vi "configureTiming.vi"(8 "error in (no error)":errorcluster, 11 "ICCameraAcquisitor in":refnum<class "ICCameraAcquisitor.lvclass">) -> (0 "error out":errorcluster, 3 "ICCameraAcquisitor out":refnum<class "ICCameraAcquisitor.lvclass">)   [LabVIEW 2009, in "Hardware.lvlib" / "Channels.lvlib" / "ICCameraAcquisitor.lvclass"]
uses:
  ICCameraAcquisitor.lvclass
  ICCameraAcquisitor.lvclass/ICCameraAcquisitor.ctl
  CameraAcquisitor.lvclass
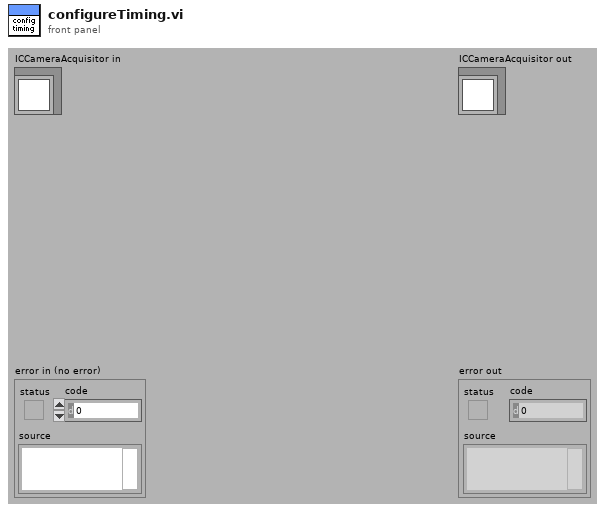
[diagram p1: front panel]
types:
  T1 = cluster{"shutter Open Time":dbl, "Shutter Close Time":dbl, "Exposure Time":dbl, " AccumulatedCycleTime":dbl, " KineticCycleTime":dbl, "Number of Accumulations":dbl, "Number in Kinetic Series ":dbl, "Shutter Mode":dbl}
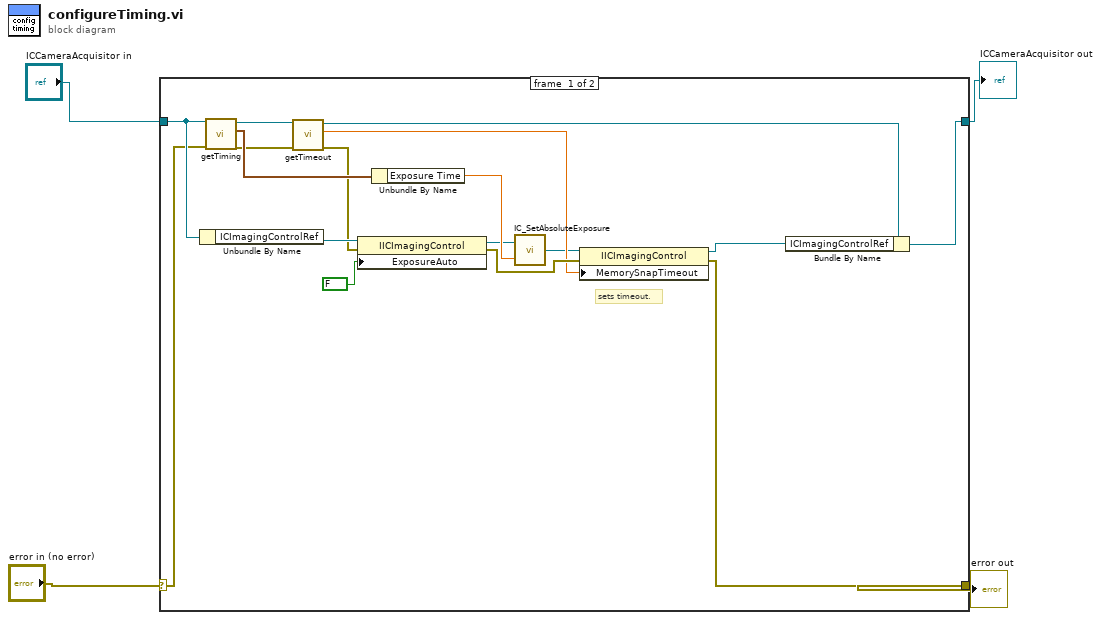
[diagram p0: block diagram]
diagram:
  n1 = case shown="No Error" "error in (no error)" {
    selector: "error in (no error)" -> [w18 w22]
    tunnel: "ICCameraAcquisitor in" -> [w19 w23]
    tunnel: [w10 w23] -> w3
    tunnel: [w14 w22] -> w1
    frame #0 {
      # "sets timeout."
      n2 = Unbundle By Name(w19) -> ("ICImagingControlRef"=w20:refnum<k7>)
      n3 = call-dynamic "getTiming.vi"("error in (no error)"=w18, "CameraAcquisitor.lvclass in"=w19) -> ("error out"=w9:errorcluster, "Timing"=w17:T1, "CameraAcquisitor.lvclass out"=w13:refnum<class "ICCameraAcquisitor.lvclass">)  [unwired: 7 in]
      n4 = call "getTimeout.vi"("error in (no error)"=w9, "CameraAcquisitor.lvclass in"=w13) -> ("error out"=w8:errorcluster, "Timeout"=w12:dbl, "CameraAcquisitor.lvclass out"=w11:refnum<class "ICCameraAcquisitor.lvclass">)  [unwired: 7 in]
      n5 = property class="IICImagingControl"(reference=w20, error in=w8, "ExposureAuto"=FALSE) -> (reference out=w5:refnum<k7>, error out=w15:errorcluster)
      n6 = Unbundle By Name(w17) -> ("Exposure Time"=w7:dbl)
      n7 = call <userlib>:"IC_SetAbsoluteExposure.vi"("Absolute Exposure Time"=w7, "ICImagingControl 4"=w5) -> ("ICImagingControl 3"=w6:refnum<k7>)
      n8 = property class="IICImagingControl"(reference=w6, error in=w15, "MemorySnapTimeout"=w12) -> (reference out=w16:refnum<k7>, error out=w14:errorcluster)
      n9 = Bundle By Name(cluster=w11, "ICImagingControlRef"=w16) -> (w10:refnum<class "ICCameraAcquisitor.lvclass">)
    }
    frame #1 {
    }
  }
  "error out" <- w1
  "ICCameraAcquisitor out" <- w3
